vi "Routine.vi"(11 "Hello World Event in":refnum<class "Hello World Event.lvclass">) -> (3 "Hello World Event out":refnum<class "Hello World Event.lvclass">)   [LabVIEW 2021, in "Hello World Event.lvlib" / "Hello World Event.lvclass"]
uses:
  Hello World Event.lvclass
  C:/Program Files/National Instruments/LabVIEW 2021/vi.lib/Nathan Davis/jettl/jettl/jettl/jettl.lvclass
  Hello World Event.lvclass/Hello World Event.ctl
  <vilib>/Nathan Davis/jettl/jettl/Event/Event.lvclass
  <vilib>/Nathan Davis/jettl/jettl/Msg Strategy/Msg Strategy.lvclass
  Hello World Msg Strategy/Hello World Msg Strategy.lvlib
  Iterate Msg Strategy/Iterate Msg Strategy.lvlib
  Auto Iterate Msg Strategy/Auto Iterate Msg Strategy.lvlib
  C:/Program Files/National Instruments/LabVIEW 2021/vi.lib/Nathan Davis/jettl/Merge Error Msg Strategy/Merge Error/Merge Error.lvclass
  C:/Program Files/National Instruments/LabVIEW 2021/vi.lib/Nathan Davis/jettl/jettl/Event/Event.lvclass
  C:/Program Files/National Instruments/LabVIEW 2021/vi.lib/Nathan Davis/jettl/jettl/Last Ack Creator Queue Msg Strategy/Last Ack Creator Queue/Last Ack Creator Queue.lvclass
  C:/Program Files/National Instruments/LabVIEW 2021/vi.lib/Nathan Davis/jettl/Override Error Msg Strategy/Override Error/Override Error.lvclass
  C:/Program Files/National Instruments/LabVIEW 2021/vi.lib/Nathan Davis/jettl/Set Panel State Msg Strategy/Set Panel State/Set Panel State.lvclass
  C:/Program Files/National Instruments/LabVIEW 2021/vi.lib/Nathan Davis/jettl/Setup Msg Strategy/Setup/Setup.lvclass
  C:/Program Files/National Instruments/LabVIEW 2021/vi.lib/Nathan Davis/jettl/Teardown Msg Strategy/Teardown/Teardown.lvclass
  C:/Users/natev/Desktop/Hello World/Hello World Event/Hello World Event/Hello World Event.lvclass
  C:/Users/natev/Desktop/Hello World/Hello World Event/Hello World Msg Strategy/Hello World/Hello World.lvclass
  C:/Users/natev/Desktop/Hello World/Hello World Event/Iterate Msg Strategy/Iterate/Iterate.lvclass
  C:/Users/natev/Desktop/Hello World/Hello World Event/Auto Iterate Msg Strategy/Auto Iterate/Auto Iterate.lvclass
panel:
  in  "Auto Iterate":bool
  in  "Iterate Once":bool
  out "Waveform Chart":dbl(graph)
  in  "Hello World String":string
  in  "Display Hello World":bool
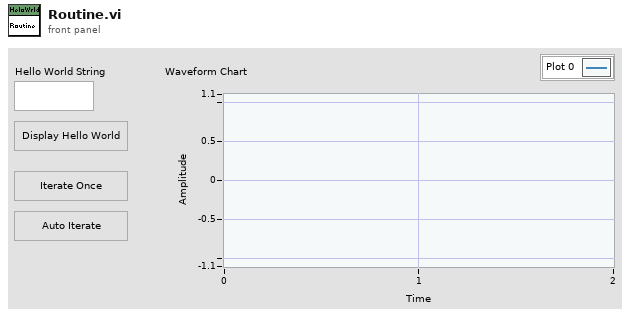
[diagram p1: front panel]
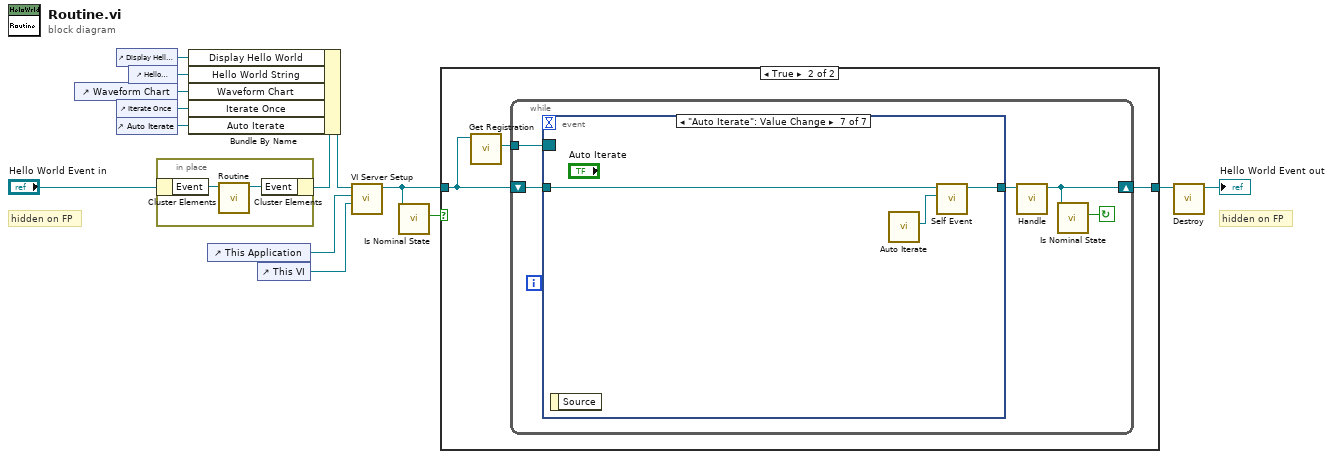
[diagram p0: block diagram]
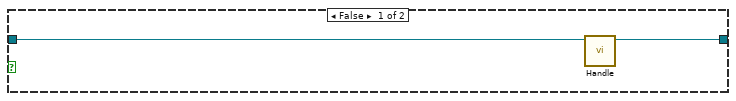
[diagram p2: hidden frame]
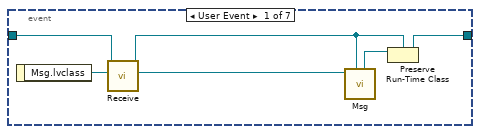
[diagram p3: hidden frame]
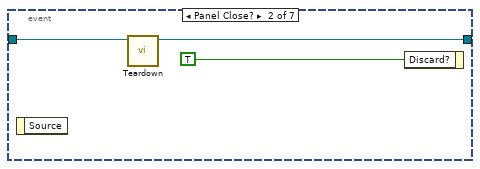
[diagram p4: hidden frame]
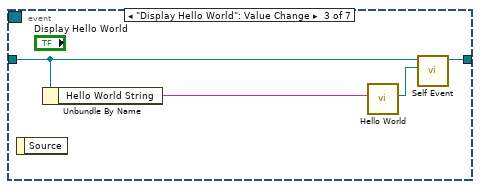
[diagram p5: hidden frame]
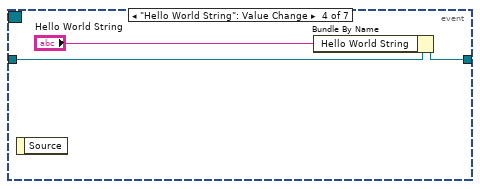
[diagram p6: hidden frame]
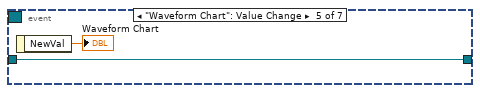
[diagram p7: hidden frame]
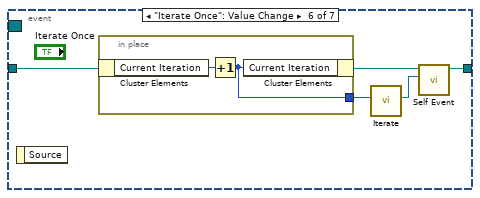
[diagram p8: hidden frame]
diagram:
  # "hidden on FP"
  # "hidden on FP"
  n1 = control-ref of="Waveform Chart"() -> (w3:refnum<vi>)
  n2 = control-ref of="Display Hello World"() -> (w5:refnum<vi>)
  n3 = control-ref of="Iterate Once"() -> (w2:refnum<vi>)
  n4 = control-ref of="Auto Iterate"() -> (w1:refnum<vi>)
  n5 = control-ref of="Hello World String"() -> (w4:refnum<vi>)
  n6 = in-place {
    n7 = in-place-cluster #1("Hello World Event in") -> ("Event"=w16:refnum<class "Event.lvclass">)
    n8 = call-dynamic "Routine.vi"("jettl in"=w16) -> ("jettl out"=w15:refnum<class "Event.lvclass">)  [unwired: 10 in]
    n9 = in-place-cluster #1("Event"=w15) -> (w9:refnum<class "Hello World Event.lvclass">)
  }
  n10 = Bundle By Name(cluster=w9, "Display Hello World"=w5, "Hello World String"=w4, "Waveform Chart"=w3, "Iterate Once"=w2, "Auto Iterate"=w1) -> (w6:refnum<class "Hello World Event.lvclass">)
  n11 = control-ref of="This Application"() -> (w8:refnum<vi>)
  n12 = control-ref of="This VI"() -> (w7:refnum<vi>)
  n13 = call-dynamic "VI Server Setup.vi"("This VI"=w7, "This Application"=w8, "Hello World Event in"=w6) -> ("Hello World Event out"=w11:refnum<class "Hello World Event.lvclass">)  [unwired: 8 in]
  n14 = call-dynamic "Is Nominal State.vi"("Hello World Event in"=w11) -> ("Is Nominal State?"=w10:bool)  [unwired: 10 in]
  n15 = case shown="True" w10 {
    tunnel: w11 -> [w18 w21]
    tunnel: [w17 w19] -> w13
    frame False {
      n16 = call-dynamic "Handle.vi"("Hello World Event in"=w18) -> ("Hello World Event out"=w17:refnum<class "Hello World Event.lvclass">)  [unwired: 10 in]
    }
    frame True {
      n17 = call-dynamic "Get Registration.vi"("Hello World Event in"=w21) -> ("Registration"=w20:refnum<event-registration>)  [unwired: 10 in]
      n18 = while {
        shift-right: [w23] -> w19
        shift-left: w21 -> [w25]
        tunnel: w20 -> [w26]
        stop <- w22 continue-if-true
        n19 = event shown="[6] \"Auto Iterate\": Value Change" {
          selector: w26 -> [_ _ _ _ _ _ _]
          dyn-events: _ -> [_ _ _ _ _ _ _]
          timeout: _ -> [_ _ _ _ _ _ _]
          tunnel: w25 -> [w30 w34 w37 w42 w44 w49 w54]
          tunnel: [w32 w33 w39 w41 w44 w48 w53] -> w24
          event User Event {
            n20 = event-data() -> ("Msg.lvclass"=w27:refnum<class "Msg Strategy.lvclass">)  [unwired: 1 in]
            n21 = call-dynamic "Receive.vi"("Msg Strategy in"=w27, "Hello World Event in"=w30) -> ("Msg Strategy out"=w28:refnum<class "Msg Strategy.lvclass">, "Hello World Event out"=w29:refnum<class "Hello World Event.lvclass">)  [unwired: 8 in]
            n22 = call-dynamic "Msg.vi"("jettl in"=w29, "Msg Strategy in"=w28) -> ("jettl out"=w31:refnum<class "jettl.lvclass">)  [unwired: 9 in]
            n23 = Preserve Run-Time Class(object in=w31, 2:w29) -> (object out=w32:refnum<class "Hello World Event.lvclass">)  [unwired: 1 in, 1 out]
          }
          event Panel Close? {
            n24 = event-data() -> ()  [unwired: 1 in, 1 out]
            n25 = call-dynamic "Teardown.vi"("Hello World Event in"=w34) -> ("Hello World Event out"=w33:refnum<class "Hello World Event.lvclass">)  [unwired: 10 in]
            n26 = event-data("Discard?"=TRUE) -> ()  [unwired: 1 in, 1 out]
          }
          event "Display Hello World": Value Change {
            n27 = event-data() -> ()  [unwired: 1 in, 1 out]
            n28 = Unbundle By Name(w37) -> ("Hello World String"=w36:string)
            n29 = call "Hello World.vi"("String"=w36) -> ("Msg Strategy"=w38:refnum<class "Msg Strategy.lvclass">)  [unwired: 10 in]
            n30 = call-dynamic "Self Event.vi"("Msg Strategy"=w38, "Hello World Event in"=w37) -> ("Hello World Event out"=w39:refnum<class "Hello World Event.lvclass">)  [unwired: 9 in]
          }
          event "Hello World String": Value Change {
            n31 = event-data() -> ()  [unwired: 1 in, 1 out]
            n32 = Bundle By Name(cluster=w42, "Hello World String"="Hello World String") -> (w41:refnum<class "Hello World Event.lvclass">)
          }
          event "Waveform Chart": Value Change {
            n33 = event-data() -> ("NewVal"=→"Waveform Chart":dbl)  [unwired: 1 in]
          }
          event "Iterate Once": Value Change {
            n34 = event-data() -> ()  [unwired: 1 in, 1 out]
            n35 = in-place {
              in-place-border: [w50] -> w45
              n36 = in-place-cluster #2(w49) -> ("Current Iteration"=w51:i32)
              n37 = Increment(x=w51) -> (x+1=w50:i32)
              n38 = in-place-cluster #2("Current Iteration"=w50) -> (w46:refnum<class "Hello World Event.lvclass">)
            }
            n39 = call "Iterate.vi"("Iterate"=w45) -> ("Msg Strategy"=w47:refnum<class "Msg Strategy.lvclass">)  [unwired: 10 in]
            n40 = call-dynamic "Self Event.vi"("Msg Strategy"=w47, "Hello World Event in"=w46) -> ("Hello World Event out"=w48:refnum<class "Hello World Event.lvclass">)  [unwired: 9 in]
          }
          event "Auto Iterate": Value Change {
            n41 = event-data() -> ()  [unwired: 1 in, 1 out]
            n42 = call "Auto Iterate.vi"() -> ("Msg Strategy"=w52:refnum<class "Msg Strategy.lvclass">)  [unwired: 11 in]
            n43 = call-dynamic "Self Event.vi"("Msg Strategy"=w52, "Hello World Event in"=w54) -> ("Hello World Event out"=w53:refnum<class "Hello World Event.lvclass">)  [unwired: 9 in]
          }
        }
        n44 = call-dynamic "Handle.vi"("Hello World Event in"=w24) -> ("Hello World Event out"=w23:refnum<class "Hello World Event.lvclass">)  [unwired: 10 in]
        n45 = call-dynamic "Is Nominal State.vi"("Hello World Event in"=w23) -> ("Is Nominal State?"=w22:bool)  [unwired: 10 in]
      }
    }
  }
  n46 = call-dynamic "Destroy.vi"("Hello World Event in"=w13) -> ("Hello World Event out"=→"Hello World Event out":refnum<class "Hello World Event.lvclass">)  [unwired: 10 in]
